vi "MAPP_StopOrExit.vi"(0 "Error In":errorcluster) -> ()   [LabVIEW 2018]
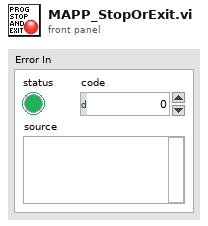
[diagram p1: front panel]
types:
  T1 = enum32{"invalid app kind", "Development System", "Run Time System", "Student Edition", "Embedded LabVIEW", "Evaluation", "Custom"}
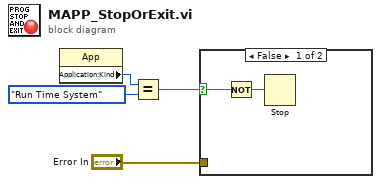
[diagram p0: block diagram]
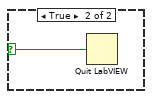
[diagram p2: hidden frame]
diagram:
  n1 = property on="Property Node" class="App"() -> ("Application:Kind"=w4:T1)  [unwired: 2 in, 2 out]
  n2 = Equal?(x=w4, y=T1."Run Time System") -> (x = y?=w2:bool)
  n3 = case shown="False" w2 {
    selector: w2 -> [w6 w7]
    tunnel: "Error In" -> [_ _]
    frame False {
      n4 = Not(x=w6) -> (.not. x?=w5:bool)
      n5 = Stop(stop? (T)=w5) -> ()
    }
    frame True {
      n6 = Quit LabVIEW(quit? (T)=w7) -> ()
    }
  }
